vi "usbPB_stop_fix.vi"(11 "1D_array_of_24ch_pb_array\nIN":cluster{"24ch_pb_array":T1}[](array[cluster]) {"24ch_pb_array"."Time (s)" min=5e-08 format="%.2p"; "24ch_pb_array"."Op Code" items=["Continue", "Stop", "Loop", "End Loop", "JSR", "RTS", "Go To", "Long Delay", "Wait"]; "24ch_pb_array"."Instruct Data" format="%#.2p"}) -> (3 "1D_array_of_24ch_pb_array\nOUT":cluster{"24ch_pb_array":T1}[](array[cluster]) {"24ch_pb_array"."Time (s)" min=5e-08 format="%.2p"; "24ch_pb_array"."Op Code" items=["Continue", "Stop", "Loop", "End Loop", "JSR", "RTS", "Go To", "Long Delay", "Wait"]; "24ch_pb_array"."Instruct Data" format="%#.2p"})   [LabVIEW 2016]
uses:
  Controls/PulseBlaster/24ch_pb_array.ctl
  Controls/PulseBlaster/24ch_single_timing_column.ctl
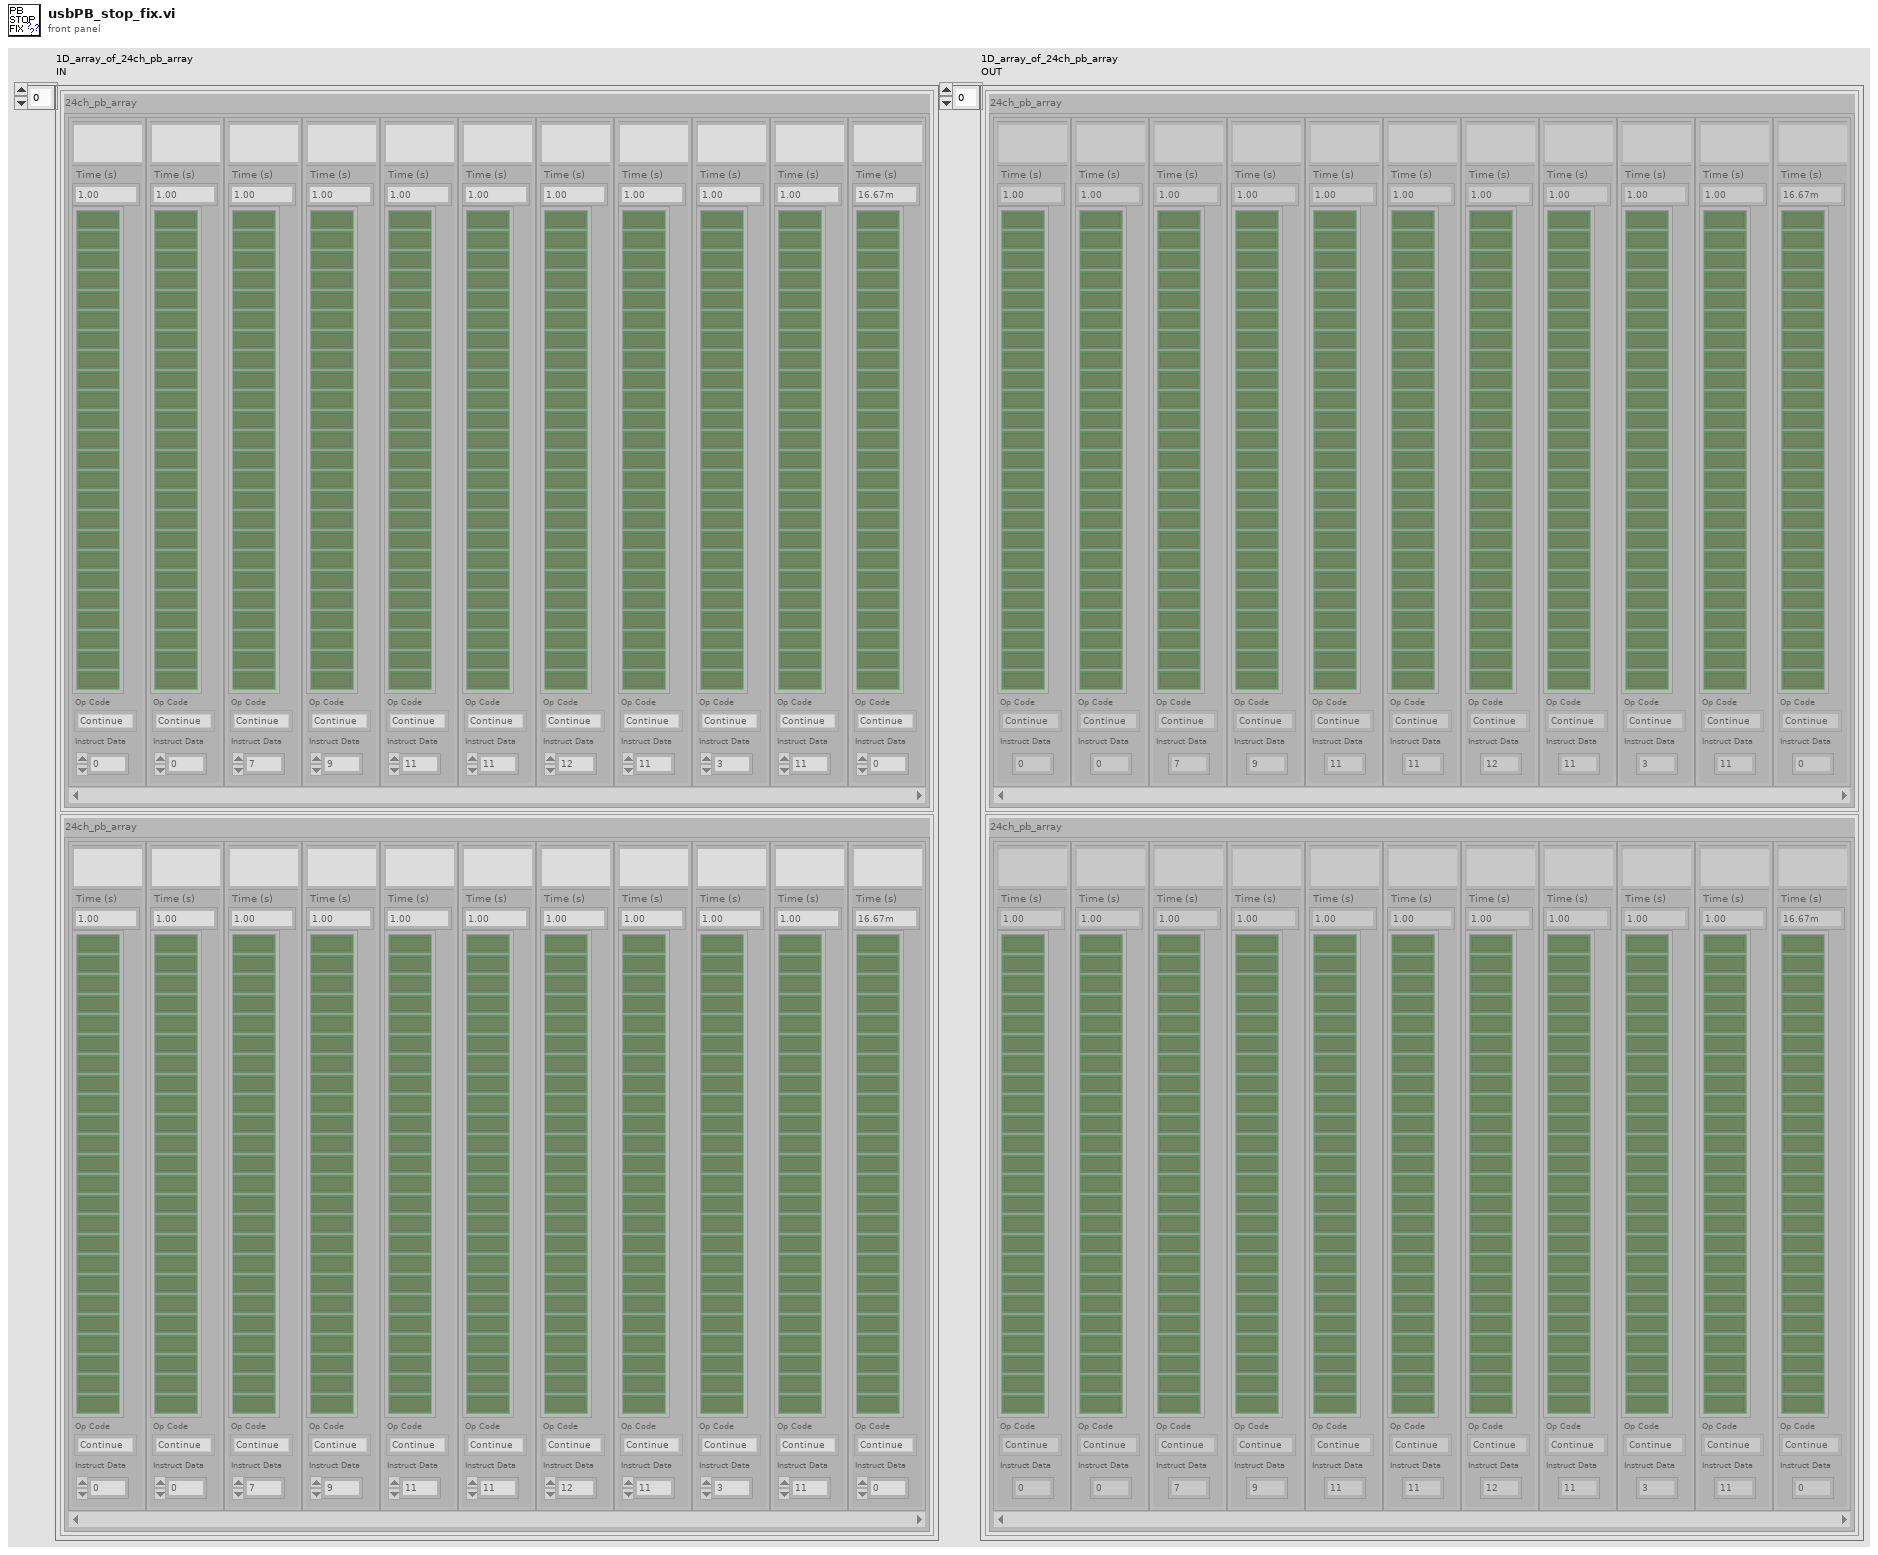
[diagram p1: front panel]
types:
  T1 = typedef "24ch_pb_array.ctl" = T2[]
  T2 = typedef "24ch_single_timing_column.ctl" = cluster{"Instruct Data":i32, "Op Code":i32, "Flags":bool[], "Comments":string, "Time (s)":dbl}
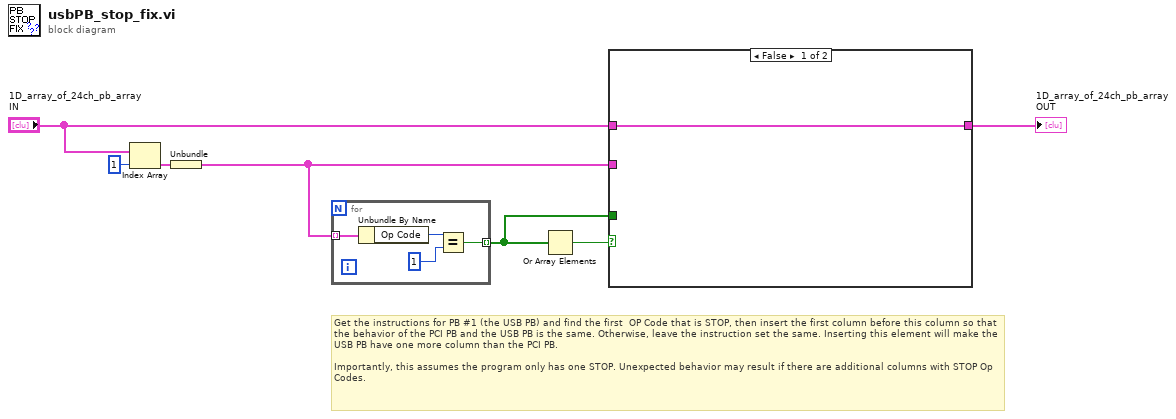
[diagram p0: block diagram]
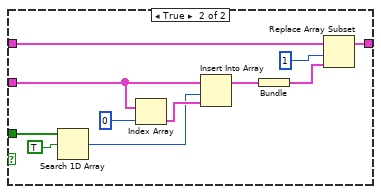
[diagram p2: hidden frame]
diagram:
  # "Get the instructions for PB #1 (the USB PB) and find the first  OP Code that is STOP, then insert the first column before this column so that the behavior of the PCI PB and the USB PB is the same. Otherwise, leave the instruction set the same. Inserting this element will make the USB PB have one more column than the PCI PB.\n\nImportantly, this assumes the program only has one STOP. Unexpected behavior may result if there are additional columns with STOP Op Codes."
  n1 = Index Array(array="1D_array_of_24ch_pb_array\nIN", index=1) -> (element=w6:cluster{"24ch_pb_array":T1})
  n2 = Unbundle(w6) -> ("24ch_pb_array"=w3:T1)
  n3 = for {
    tunnel: w3 -> [w11] mode=indexing
    tunnel: [w8] -> w1 mode=indexing
    n4 = Unbundle By Name(w11) -> ("Op Code"=w10:i32)
    n5 = Equal?(x=w10, y=1) -> (x = y?=w8:bool)
  }
  n6 = Or Array Elements(Boolean array=w1) -> (logical OR=w2:bool)
  n7 = case shown="False" w2 {
    tunnel: "1D_array_of_24ch_pb_array\nIN" -> [w12 w23]
    tunnel: [w12 w22] -> w4
    tunnel: w3 -> [_ w16]
    tunnel: w1 -> [_ w15]
    frame False {
    }
    frame True {
      n8 = Search 1D Array(1D array=w15, element=TRUE) -> (index of element=w13:i32)  [unwired: 1 in]
      n9 = Index Array(array=w16, index=0) -> (element=w20:T2)
      n10 = Insert Into Array(array=w16, index=w13, new element=w20) -> (w19:T1)
      n11 = Bundle("24ch_pb_array"=w19) -> (w18:cluster{"24ch_pb_array":T1})  [unwired: 1 in]
      n12 = Replace Array Subset(array=w23, new element=w18, index=1) -> (w22:cluster{"24ch_pb_array":T1}[])
    }
  }
  "1D_array_of_24ch_pb_array\nOUT" <- w4
